vi "Create Cmd Queue.vi"(8 "error in (no error)":errorcluster, 11 "FTP in":refnum<class "FTP.lvclass">) -> (0 "error out":errorcluster, 3 "FTP out":refnum<class "FTP.lvclass">)   [LabVIEW 2020, in "FTP.lvlib" / "FTP.lvclass"]
uses:
  FTP.lvclass
  FTP.lvclass/FTP.ctl
  controls/CmdCluster.ctl
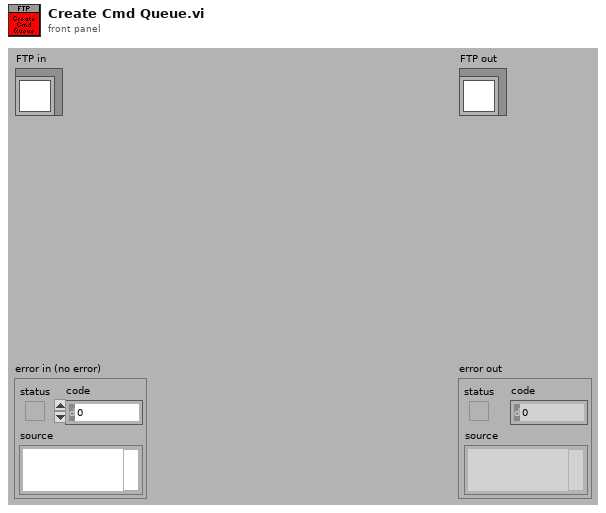
[diagram p1: front panel]
types:
  T1 = typedef "FTP.lvlib/FTP.lvclass/CmdCluster.ctl" = cluster{"CmdSting":string, "FromClient":bool}
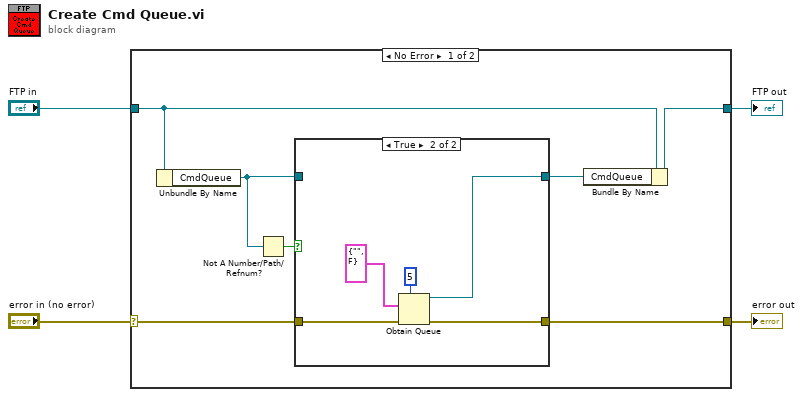
[diagram p0: block diagram]
diagram:
  n1 = case shown="No Error" "error in (no error)" {
    selector: "error in (no error)" -> [w9 w20]
    tunnel: [w8 w20] -> w3
    tunnel: [w11 w19] -> w1
    tunnel: "FTP in" -> [w7 w19]
    frame No Error {
      n2 = Unbundle By Name(w7) -> ("CmdQueue"=w5:refnum<queue>)
      n3 = Not A Number/Path/Refnum?(number/path/refnum=w5) -> (NaN/Path/Refnum?=w6:bool)
      n4 = case shown="True" w6 {
        tunnel: [w12 w16] -> w10
        tunnel: w9 -> [w13 w15]
        tunnel: [w13 w14] -> w8
        tunnel: w5 -> [w12 _]
        frame False {
        }
        frame True {
          n5 = Obtain Queue(max queue size (-1, unlimited)=5, element data type=T1 {"CmdSting"="", "FromClient"=FALSE} ("CmdCluster"), error in (no error)=w15) -> (queue out=w16:refnum<queue>, error out=w14:errorcluster)  [unwired: 2 in, 1 out]
        }
      }
      n6 = Bundle By Name(cluster=w7, "CmdQueue"=w10) -> (w11:refnum<class "FTP.lvclass">)
    }
    frame Error {
    }
  }
  "error out" <- w3
  "FTP out" <- w1
